vi "Assembly Type.vi"(0 "Assembly Run.lvclass In":refnum<class "Assembly Run.lvclass">) -> (4 "Assembly Run.lvclass Out":refnum<class "Assembly Run.lvclass">, 6 "Geometry":enum16{"Full", "Right Partial"}(ring), 8 "Density":enum16{"LD", "HD"}(ring), 10 "Sensor Size":enum16{"120", "200", "300"}(ring), 15 "Component to add":enum16{"Sensor", "Hexaboard"}(ring))   [LabVIEW 2021, in "Assembly Run.lvclass"]
uses:
  Assembly Run.lvclass
  <vilib>/JDP Science/JDP Science Common Utilities/JDP Utility.lvlib
panel:
  in  "stop":bool
  in  "Component to add In":enum16{"Sensor", "Hexaboard"}(ring)
  in  "Sensor Size In":enum16{"120", "200", "300"}(ring)
  in  "Density In":enum16{"LD", "HD"}(ring)
  in  "Geometry In":enum16{"Full", "Right Partial"}(ring)
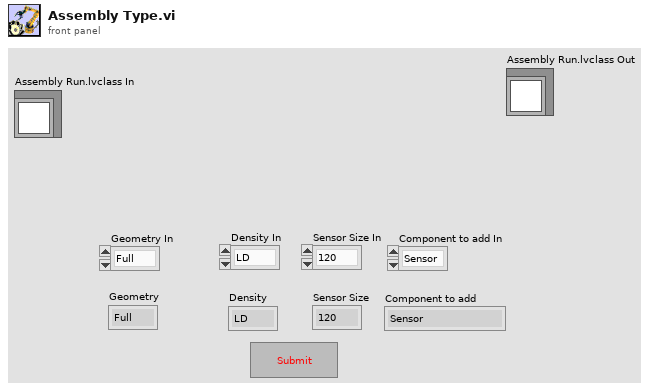
[diagram p1: front panel]
types:
  T1 = typedef "File Paths.ctl" = cluster{"Glue Pattern Folder":path, "Carrier Tray Folder":path, "Pick Up Tool Fixture Folder":path, "Components Folder":path, "Bellows Tool Offset.txt":path, "Pick Up Tool Offset.txt":path, "Dispense Tip Offset.txt":path, "Log Files":path, "Gantry Assembly Map.txt":path, "Syringe and offset map.txt":path, "Controllers Folder":path}
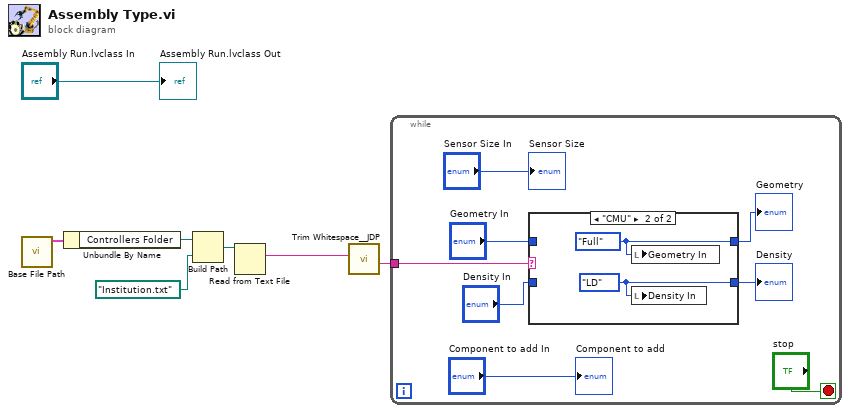
[diagram p0: block diagram]
diagram:
  n1 = call "Base File Path.vi"() -> ("Paths Out"=w7:T1)  [unwired: 11 in]
  n2 = Unbundle By Name(w7) -> ("Controllers Folder"=w6:path)
  n3 = Build Path(base path=w6, name or relative path=path "Institution.txt") -> (appended path=w4:path)
  n4 = Read from Text File(file (use dialog)=w4) -> (text=w2:string)  [unwired: 3 in, 3 out]
  n5 = call <vilib>:"Trim Whitespace__JDP.vi"("String in"=w2) -> ("String out"=w1:string)  [unwired: 6 in]
  n6 = while {
    tunnel: w1 -> [w12]
    stop <- "stop" stop-if-true
    n7 = case shown="\"CMU\"" w12 {
      tunnel: "Geometry In" -> [w17 _]
      tunnel: [w17 w19] -> w9
      tunnel: "Density In" -> [w16 _]
      tunnel: [w16 w18] -> w11
      frame "UCSB", Default {
      }
      frame "CMU" {
        w18 = enum16{"LD", "HD"}."LD" ("Density")
        w19 = enum16{"Full", "Right Partial"}."Full" ("Geometry")
        n8 = local write "Geometry In"(w19) -> ()
        n9 = local write "Density In"(w18) -> ()
      }
    }
    "Density" <- w11
    "Geometry" <- w9
    "Sensor Size" <- "Sensor Size In"
    "Component to add" <- "Component to add In"
  }
  "Assembly Run.lvclass Out" <- "Assembly Run.lvclass In"
